vi "New Instrumentation 2021.vi"() -> ()   [LabVIEW 2021]
uses:
  <vilib>/Analysis/NI_AALBase.lvlib
  <vilib>/Analysis/baseanly.llb/Mean (DBL).vi
panel:
  in  "Array":dbl[](array[numeric])
  in  "file name":string
  in  "file path":path
  out "Pre-Combustion Chamber: Temperature":dbl(graph)
  out "Run Tank: Temperature":dbl(graph)
  out "Run Tank: Pressure":dbl(graph)
  out "N20 Post-Tank: Pressure":dbl(graph)
  out "N2 Post-tank: Pressure":dbl(graph)
  out "Stream Parameters":T1 {"Device Backlog [%]" format="%.2f"}
  in  "PC buffer size (seconds)":dbl=10.0 format="%.2f"
  in  "Scan List (-)":u8[](array[numeric])=[31, 31, 31, 31, 31, 31, 31, 31, 31, 31, 31, 31, 31, 31, 31, 31, 31, 31, 31, 31, 31, 31, 31, 31, 31, 31, 31, 31, 31, 31, 31, 31, 31, 31, 31, 31, 31, 31, 31, 31, 31, 31, 31, 31, 31, 31, 31, 31, 31, 31, 31, 31, 31, 31, 31, 31, 31, 31, 31, 31, 31, 31, 31, 31, 31, 31, 31, 31, 31, 31, 31, 31, 31, 31, 31, 31, 31, 31, 31, 31, 31, 31, 31, 31, 31, 31, 31, 31, 31, 31, 31, 31, 31, 31, 31, 31, 31, 31, 31, 31, 31, 31, 31, 31, 31, 31, 31, 31, 31, 31, 31, 31, 31, 31, 31, 31, 31, 31, 31, 31, 31, 31, 31, 31, 31, 31, 31, 31]
  out "Data":dbl[][](array[numeric]) format="%.3f"
  in  "Scan List (+)":u8[](array[numeric])=[0, 1, 2, 3]
  out "# of iterations":i32
  in  "Scan Rate (Hz)":dbl=1000.0 format="%.3f"
  in  "stop":bool
  out "Error Message":string
  # "File Save Location:"
  # "This example streams from the first found USB U3.  Streaming\nrequires U3 hardware revision 1.21+."
  # "The + scan list is the positive\nchannels.  For each element in\nthe + list, there must also be\nan element in the - list, which is\nthe negative channels.  For\nsingle-ended channels, put in\n31 for the negative channel.\n\nTo remove an element, right-click\non it, select Data Operations =>\nRemove Element.\n\nTo empty an array, right-click\nnear the edge, select Data\nOperations => Empty Array.\n\nOther useful operations:  From the\nOperate menu are \"Make Current\nValues Default\" and \"Reinitialize\nTo Default\"."
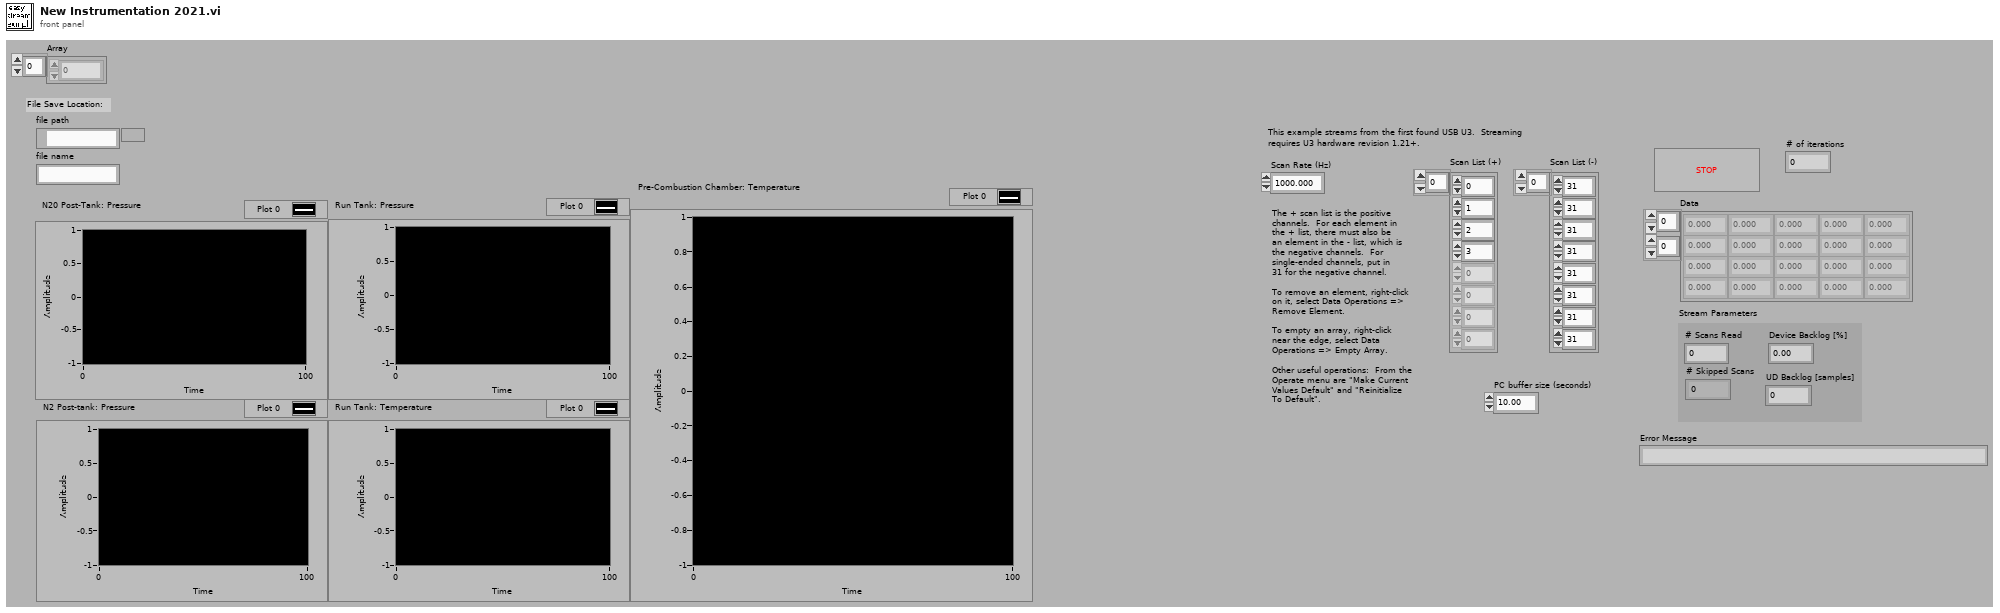
[diagram p1: front panel]
types:
  T1 = cluster{"# Scans Read":i32, "# Skipped Scans":i32, "Device Backlog [%]":dbl, "UD Backlog [samples]":i32}
  T2 = enum16{"open", "open or create", "create or replace", "create", "open (read-only)"}
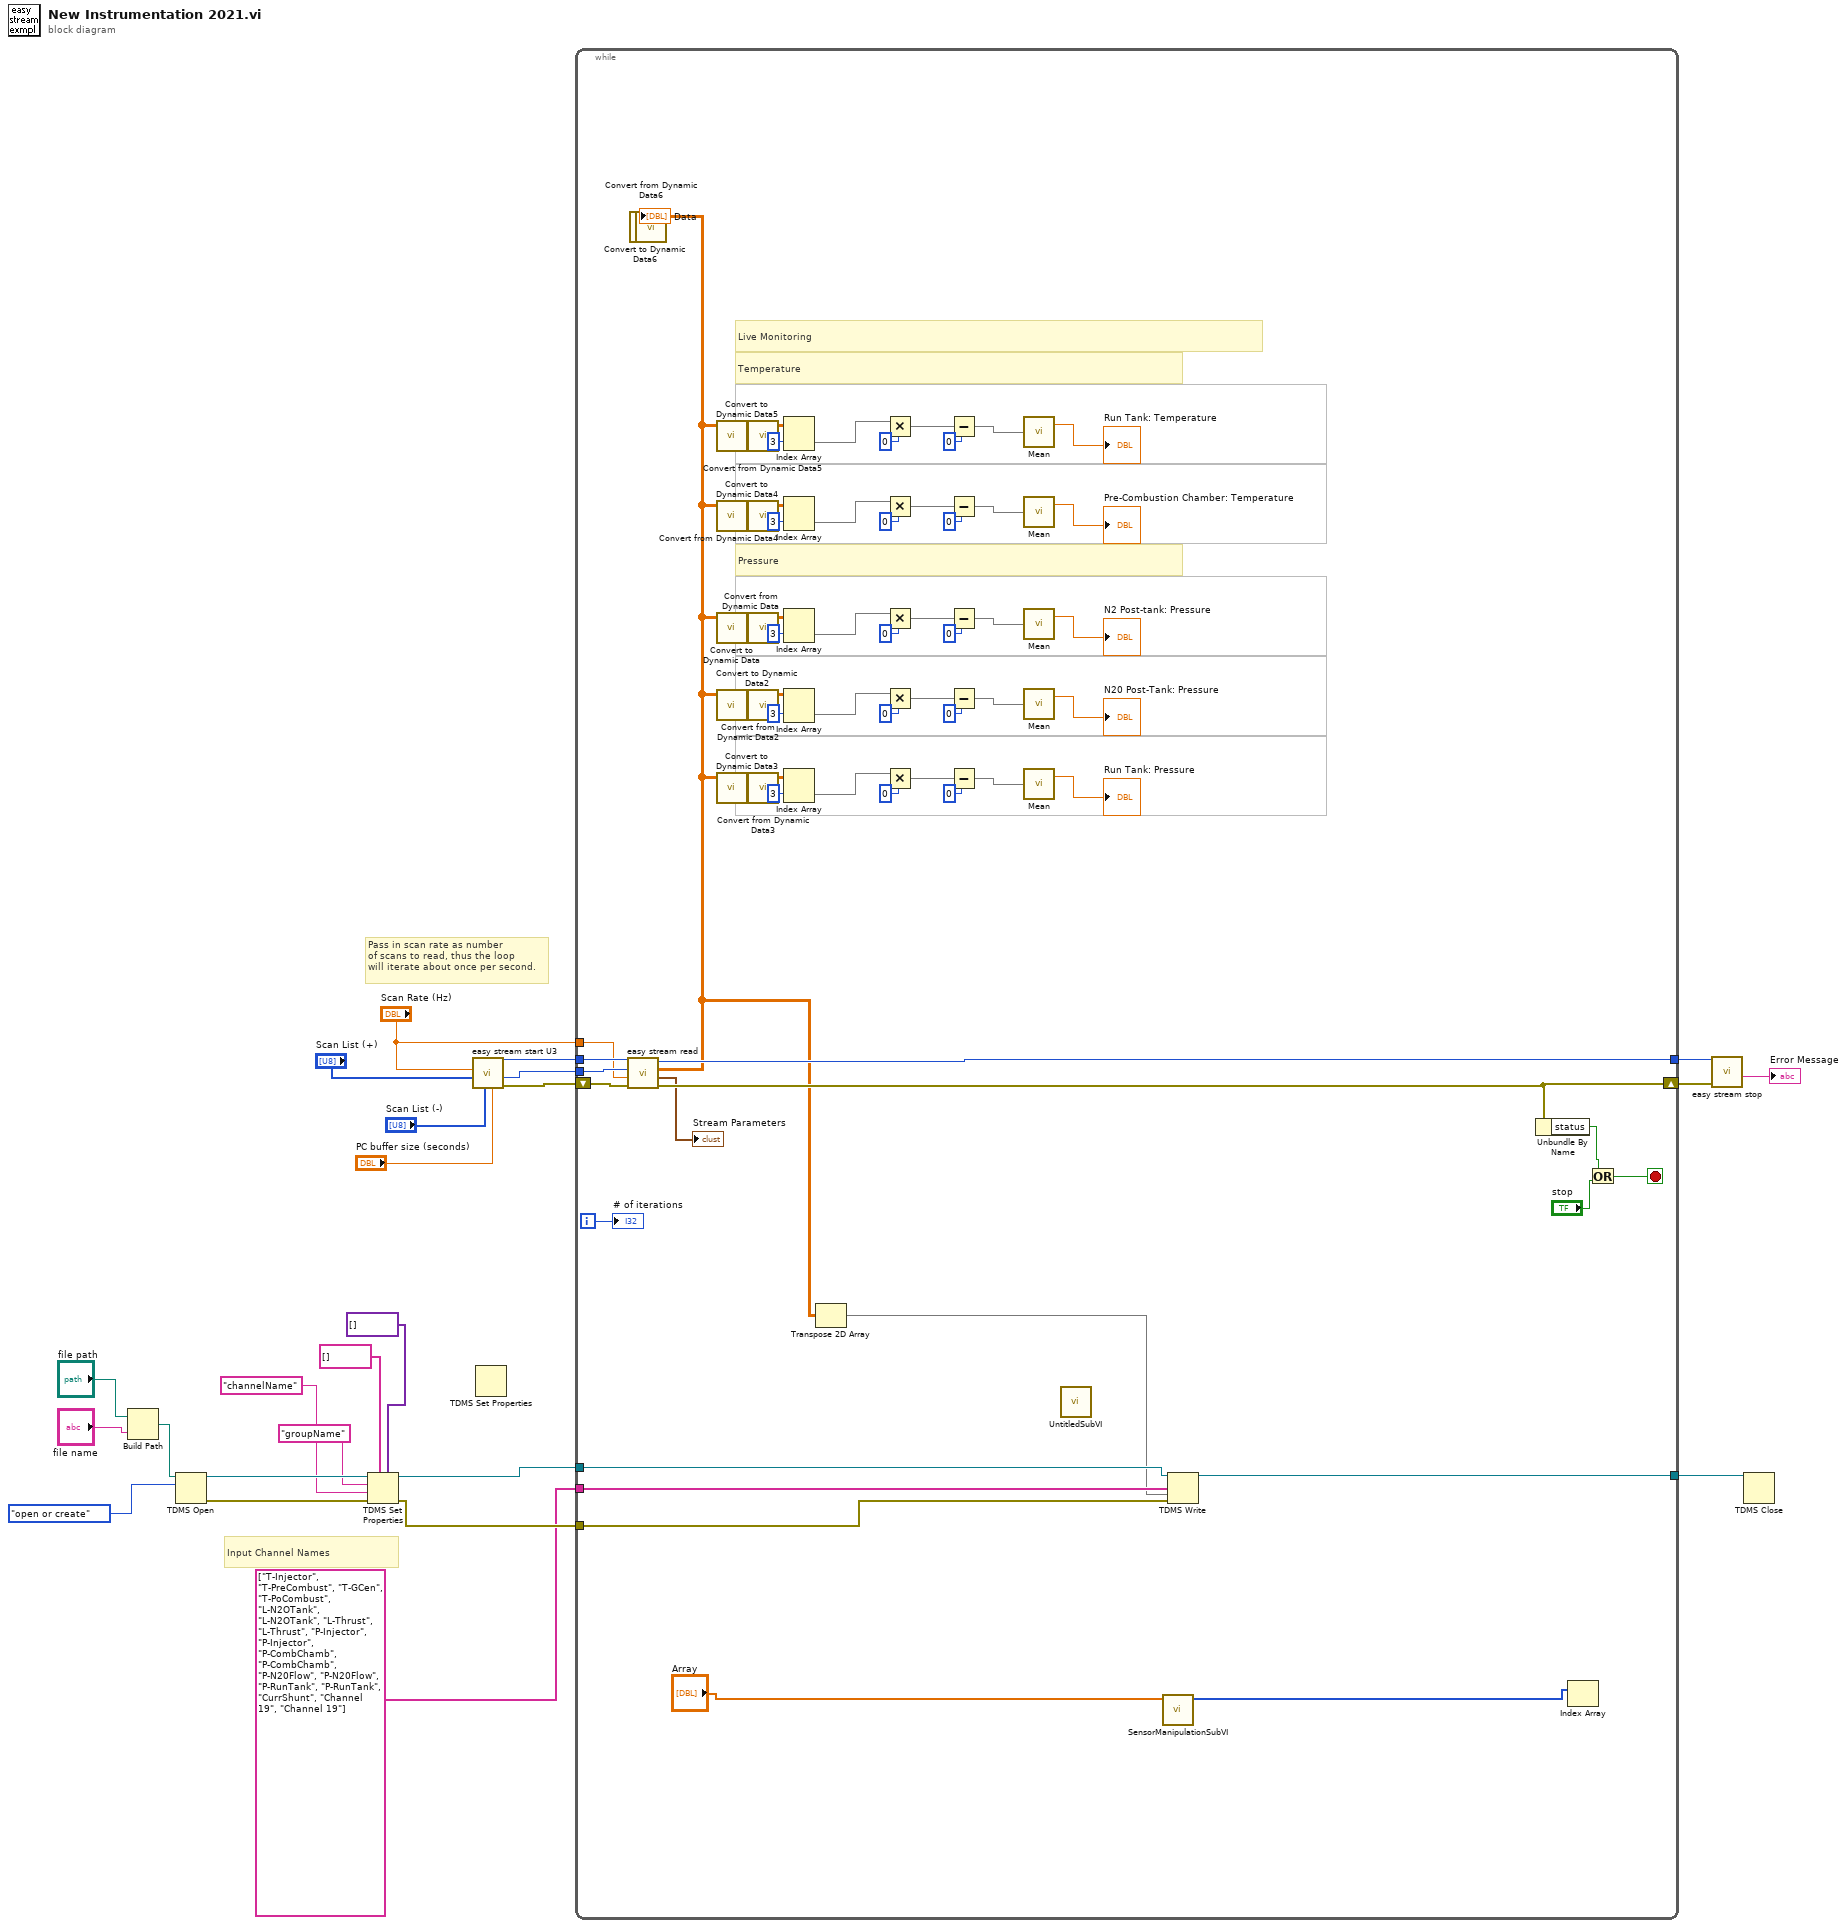
[diagram p0: block diagram]
diagram:
  # "Input Channel Names"
  # "Pass in scan rate as number\nof scans to read, thus the loop\nwill iterate about once per second."
  n1 = Build Path(base path="file path", name or relative path="file name") -> (appended path=w7:path)
  n2 = TDMS Open(10:T2."open or create" ("operation (0:open)"), 11:w7) -> (0:w14:errorcluster, 3:w13:refnum<k34>)  [unwired: 5 in]
  n3 = TDMS Set Properties(5:variant[] [] ("property values"), 7:string[] [] ("property names"), 8:w14, 9:"channelName" ("channel name"), 10:"groupName" ("group name"), 11:w13) -> (0:w12:errorcluster, 3:w11:refnum<k34>)  [unwired: 2 out]
  n4 = call "easy stream start U3.vi"("PC buffer size (seconds)"="PC buffer size (seconds)", "Scan List (-)"="Scan List (-)", "Scan List (+)"="Scan List (+)", "Scan Rate (Hz)"="Scan Rate (Hz)") -> ("error out"=w24:errorcluster, "# Channels"=w22:i32, "Handle Out"=w21:i32)  [unwired: 4 in, 1 out]
  n5 = TDMS Set Properties() -> ()  [unwired: 6 in, 4 out]
  n6 = while {
    tunnel: "Scan Rate (Hz)" -> [w81]
    tunnel: [w83] -> w19
    tunnel: w21 -> [w84]
    tunnel: w22 -> [w85]
    shift-left: w24 -> [w86]
    shift-right: [w82] -> w20
    tunnel: w12 -> [w44]
    tunnel: w11 -> [w42]
    tunnel: string[] ["T-Injector", "T-PreCombust", "T-GCen", "T-PoCombust", "L-N2OTank", "L-N2OTank", "L-Thrust", "L-Thrust", "P-Injector", "P-Injector", "P-CombChamb", "P-CombChamb", "P-N20Flow", "P-N20Flow", "P-RunTank", "P-RunTank", "CurrShunt", "Channel 19", "Channel 19"] -> [w43]
    tunnel: [w27] -> w1
    i -> [w87]
    stop <- w88 stop-if-true
    (unwired) 0.0 ("N2 Post-tank: Pressure")
    # "Temperature"
    # "Live Monitoring"
    # "Pressure"
    n7 = call "easy stream read.vi"("error in"=w86, "Scans To Read"=w81, "# Channels In Stream"=w85, "Handle In"=w84) -> ("error out"=w82:errorcluster, "Stream Parameters"=→"Stream Parameters":T1, "Data"=w29:dbl[][], "Handle Out"=w83:i32)  [unwired: 4 in]
    n8 = call "Convert to Dynamic Data6"("2D Array"=w29) -> ("Dynamic Data Type"=w30:dynamicdata)  [unwired: 3 in]
    n9 = call "Convert from Dynamic Data6"("Dynamic Data Type"=w30) -> ("Array"=→"Data":dbl[][])  [unwired: 3 in]
    n10 = call "Convert to Dynamic Data5"("2D Array"=w29) -> ("Dynamic Data Type"=w31:dynamicdata)  [unwired: 3 in]
    n11 = call "Convert to Dynamic Data4"("2D Array"=w29) -> ("Dynamic Data Type"=w32:dynamicdata)  [unwired: 3 in]
    n12 = call "Convert to Dynamic Data"("2D Array"=w29) -> ("Dynamic Data Type"=w35:dynamicdata)  [unwired: 3 in]
    n13 = call "Convert to Dynamic Data2"("2D Array"=w29) -> ("Dynamic Data Type"=w34:dynamicdata)  [unwired: 3 in]
    n14 = call "Convert to Dynamic Data3"("2D Array"=w29) -> ("Dynamic Data Type"=w33:dynamicdata)  [unwired: 3 in]
    n15 = call "Convert from Dynamic Data5"("Dynamic Data Type"=w31) -> ("Array"=w37:dbl[][])  [unwired: 3 in]
    n16 = call "Convert from Dynamic Data4"("Dynamic Data Type"=w32) -> ("Array"=w38:dbl[][])  [unwired: 3 in]
    n17 = call "Convert from Dynamic Data"("Dynamic Data Type"=w35) -> ("Array"=w41:dbl[][])  [unwired: 3 in]
    n18 = call "Convert from Dynamic Data2"("Dynamic Data Type"=w34) -> ("Array"=w40:dbl[][])  [unwired: 3 in]
    n19 = call "Convert from Dynamic Data3"("Dynamic Data Type"=w33) -> ("Array"=w39:dbl[][])  [unwired: 3 in]
    n20 = Index Array(array=w37, index (col)=3) -> (element=w52:dbl[])  [unwired: 1 in]
    n21 = Index Array(array=w38, index (col)=3) -> (element=w45:dbl[])  [unwired: 1 in]
    n22 = Index Array(array=w41, index (col)=3) -> (element=w73:dbl[])  [unwired: 1 in]
    n23 = Index Array(array=w40, index (col)=3) -> (element=w66:dbl[])  [unwired: 1 in]
    n24 = Index Array(array=w39, index (col)=3) -> (element=w59:dbl[])  [unwired: 1 in]
    n25 = Transpose 2D Array(2D array=w29) -> (transposed array=w28:dbl[][])
    n26 = Multiply(x=w52, y=0) -> (x*y=w55:dbl[])
    n27 = Multiply(x=w45, y=0) -> (x*y=w48:dbl[])
    n28 = Multiply(x=w73, y=0) -> (x*y=w76:dbl[])
    n29 = Multiply(x=w66, y=0) -> (x*y=w69:dbl[])
    n30 = Multiply(x=w59, y=0) -> (x*y=w62:dbl[])
    n31 = Subtract(x=w55, y=0) -> (x-y=w54:dbl[])
    n32 = Subtract(x=w48, y=0) -> (x-y=w47:dbl[])
    n33 = Subtract(x=w76, y=0) -> (x-y=w75:dbl[])
    n34 = Subtract(x=w69, y=0) -> (x-y=w68:dbl[])
    n35 = Subtract(x=w62, y=0) -> (x-y=w61:dbl[])
    n36 = call-poly <vilib>:"Mean.vi"("X"=w54) -> ("mean"=→"Run Tank: Temperature":dbl)  [unwired: 1 out]
    n37 = call-poly <vilib>:"Mean.vi"("X"=w47) -> ("mean"=→"Pre-Combustion Chamber: Temperature":dbl)  [unwired: 1 out]
    n38 = call-poly <vilib>:"Mean.vi"("X"=w75) -> ("mean"=→"N2 Post-tank: Pressure":dbl)  [unwired: 1 out]
    n39 = call-poly <vilib>:"Mean.vi"("X"=w68) -> ("mean"=→"N20 Post-Tank: Pressure":dbl)  [unwired: 1 out]
    n40 = call-poly <vilib>:"Mean.vi"("X"=w61) -> ("mean"=→"Run Tank: Pressure":dbl)  [unwired: 1 out]
    n41 = call "UntitledSubVI.vi"() -> ()  [unwired: 12 in]
    n42 = call "SensorManipulationSubVI.vi"("Array in"="Array") -> ("Array out"=w25:i32[])  [unwired: 10 in]
    n43 = TDMS Write(0:w42, 7:w43, 9:w28, 11:w44) -> (4:w27:refnum<k34>)  [unwired: 2 in, 3 out]
    n44 = Unbundle By Name(w82) -> ("status"=w89:bool)
    n45 = Index Array(array=w25) -> ()  [unwired: 1 in, 1 out]
    n46 = Or(x=w89, y="stop") -> (x .or. y?=w88:bool)
    "# of iterations" <- w87
  }
  n47 = call "easy stream stop.vi"("error in"=w20, "Handle In"=w19) -> ("Error Message"=→"Error Message":string)  [unwired: 7 in, 2 out]
  n48 = TDMS Close(11:w1) -> ()  [unwired: 1 in, 2 out]
